vi "LED Spikes.vi"(0 "Tote in front LED":bool, 1 "Tote inside LED":bool, 2 "Camera LED":bool, 3 "Mode":enum8{"Start", "Run", "Finish"}(ring)) -> ()   [LabVIEW 2014]
uses:
  <vilib>/Rock Robotics/SystemInterfaces/DIO/FPGA_DIORelayChannel.ctl
  <vilib>/Rock Robotics/WPI/Relay/WPI_RelayDirection.ctl
  <vilib>/Rock Robotics/WPI/Relay/WPI_RelayValue.ctl
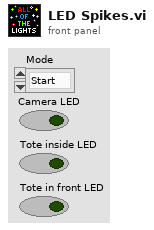
[diagram p1: front panel]
types:
  T1 = typedef "FPGA_DIORelayChannel.ctl" = enum8{"Relay 0", "Relay 1", "Relay 2", "Relay 3", "Invalid"}
  T2 = typedef "WPI_RelayDirection.ctl" = enum16{"Both directions", "Forward only", "Reverse only"}
  T3 = typedef "WPI_RelayValue.ctl" = enum16{"Off", "On", "Forward", "Reverse"}
  T4 = typedef "WPI_RelayDevRef.ctl" = cluster{"DevStatus":errorcluster, "Relay Channel":T1, "Controller":T5, "Relay Direction":T2}
  T5 = typedef "FPGA_TypedefDigitalModule.ctl" = enum16{"Controller 1"}
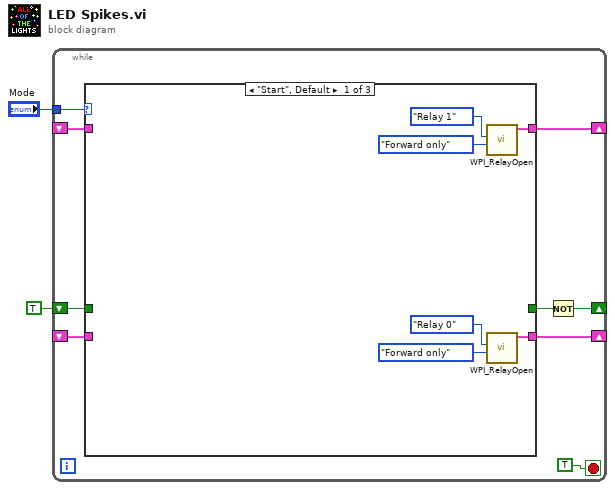
[diagram p0: block diagram]
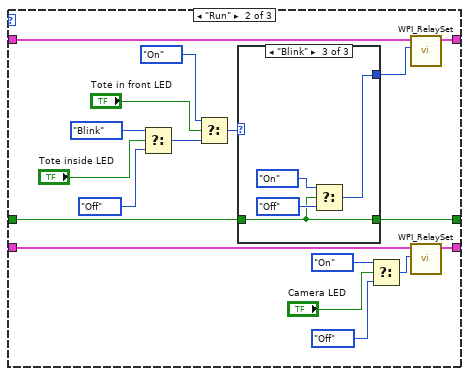
[diagram p2: hidden frame]
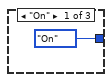
[diagram p3: hidden frame]
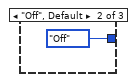
[diagram p4: hidden frame]
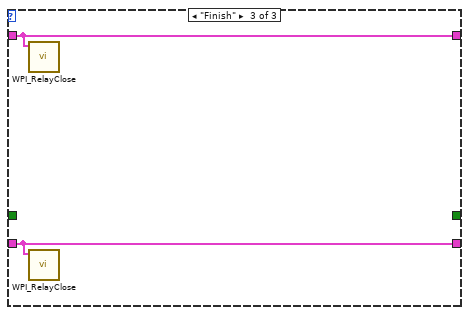
[diagram p5: hidden frame]
diagram:
  n1 = while {
    tunnel: "Mode" -> [w10]
    shift-right: [w9] -> _
    shift-left: _ -> [w8]
    shift-right: [w7] -> _
    shift-left: _ -> [w6]
    shift-right: [w3] -> _
    shift-left: TRUE ("s") -> [w5]
    stop <- TRUE stop-if-true
    n2 = case shown="\"Start\", Default" w10 {
      tunnel: [w15 w34 w43] -> w9
      tunnel: w8 -> [_ w35 w43]
      tunnel: [w12 w32 w42] -> w7
      tunnel: w6 -> [_ w33 w42]
      tunnel: w5 -> [_ w29 _]
      tunnel: [_ w30 _] -> w4
      frame "Start", Default {
        n3 = call <vilib>:"WPI_RelayOpen.vi"("Relay Direction"=WPI_RelayDirection."Forward only" ("RelayDirection"), "Relay Channel"=FPGA_DIORelayChannel."Relay 1" ("RelayChannel")) -> ("RelayDevRef"=w15:T4)  [unwired: 2 in, 7 out]
        n4 = call <vilib>:"WPI_RelayOpen.vi"("Relay Direction"=WPI_RelayDirection."Forward only" ("RelayDirection"), "Relay Channel"=FPGA_DIORelayChannel."Relay 0" ("RelayChannel")) -> ("RelayDevRef"=w12:T4)  [unwired: 2 in, 7 out]
      }
      frame "Run" {
        n5 = Select(t=enum16{"On", "Off", "Blink"}."Blink" ("ON/OFF"), s="Tote inside LED", f=enum16{"On", "Off", "Blink"}."Off" ("ON/OFF")) -> (s? t:f=w21:enum16{"On", "Off", "Blink"})
        n6 = Select(t=enum16{"On", "Off", "Blink"}."On", s="Tote in front LED", f=w21) -> (s? t:f=w19:enum16{"On", "Off", "Blink"})
        n7 = case shown="\"Blink\"" w19 {
          tunnel: [WPI_RelayValue."On" ("RelayValue") WPI_RelayValue."Off" ("RelayValue") w39] -> w31
          tunnel: w29 -> [_ _ w38]
          tunnel: [_ _ w38] -> w30
          frame "On" {
          }
          frame "Off", Default {
          }
          frame "Blink" {
            n8 = Select(t=WPI_RelayValue."On" ("RelayValue"), s=w38, f=WPI_RelayValue."Off" ("RelayValue")) -> (s? t:f=w39:T3)
          }
        }
        n9 = Select(t=WPI_RelayValue."On" ("RelayValue"), s="Camera LED", f=WPI_RelayValue."Off" ("RelayValue")) -> (s? t:f=w27:T3)
        n10 = call <vilib>:"WPI_RelaySet.vi"("RelayValue"=w31, "RelayDevRef"=w35) -> ("RelayDevRef"=w34:T4)  [unwired: 1 in, 8 out]
        n11 = call <vilib>:"WPI_RelaySet.vi"("RelayValue"=w27, "RelayDevRef"=w33) -> ("RelayDevRef"=w32:T4)  [unwired: 1 in, 8 out]
      }
      frame "Finish" {
        n12 = call <vilib>:"WPI_RelayClose.vi"("RelayDevRef"=w43) -> ()  [unwired: 1 in, 10 out]
        n13 = call <vilib>:"WPI_RelayClose.vi"("RelayDevRef"=w42) -> ()  [unwired: 1 in, 10 out]
      }
    }
    n14 = Not(x=w4) -> (.not. x?=w3:bool)
  }
